vi "test_data-type-2.vi"() -> ()   [LabVIEW 2019]
panel:
  in  "h range":cluster{i16, i16}(slide)={0, 9} scale=-180.0..180.0
  out "Numeric":i32
  in  "v range":cluster{i8, i8}(slide)={0, 9} scale=-15.0..15.0
  in  "stop":bool
  out "XY Graph":cluster{"X":dbl, "Y":dbl}[](graph)=[{"X"=0.0, "Y"=0.0}, {"X"=-0.6812582743119884, "Y"=0.18190555934279554}]
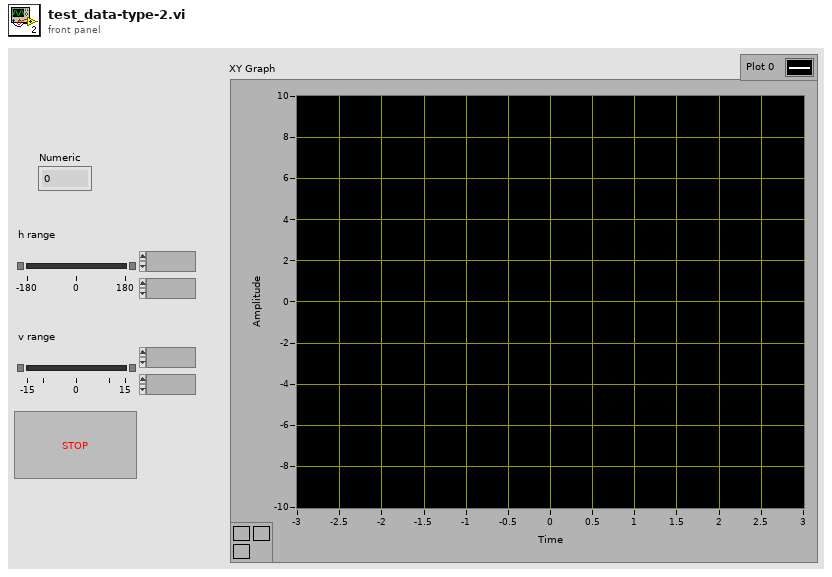
[diagram p1: front panel]
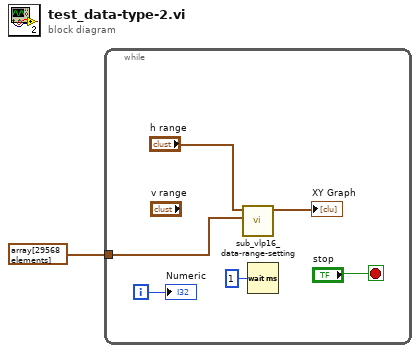
[diagram p0: block diagram]
diagram:
  n1 = while {
    tunnel: cluster{"x":dbl, "y":dbl, "z":dbl}[] array[29568 elements] ("Array") -> [w7]
    i -> [w4]
    stop <- "stop" stop-if-true
    n2 = call "sub_vlp16_data-range-setting.vi"("Array in"=w7, "min"="h range") -> ("Array out"=→"XY Graph":cluster{"x":dbl, "y":dbl}[])  [unwired: 9 in]
    n3 = Wait (ms)(milliseconds to wait=u32 1) -> ()  [unwired: 1 out]
    "Numeric" <- w4
  }
